vi "Perform_Math_Main.vi"(0 "Input_1":dbl caption="Input1", 5 "Input_2":dbl caption="Input2", 11 "Error_In":errorcluster) -> (4 "Output":dbl, 15 "Error_Out":errorcluster)   [LabVIEW 2023]
doc: "This is the main vi which Performs Math calculations using CDLL and .Net DLL."
uses:
  Controls/Operation.ctl
  Controls/DLL_Type.ctl
  D:/Project Git file/Assignments/Assignment-11/Assignment-11_LV23V/Build_.Net_Dll/Perform_Math_Assembly.dll
  Build_.Net_Dll/Perform_Math_Assembly.dll
  Build_Dll/Perform_Math.dll
panel:
  in  "DLL_Type":T1
  in  "Operation":T2
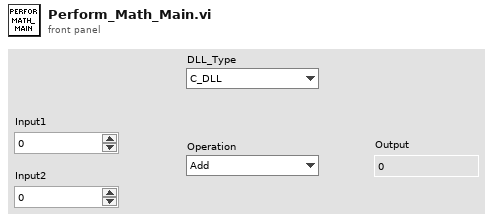
[diagram p1: front panel]
types:
  T1 = typedef "DLL_Type.ctl" = enum16{"C_DLL", ".NET_DLL"}
  T2 = typedef "Operation.ctl" = enum16{"Add", "Sub", "Mul", "Div"}
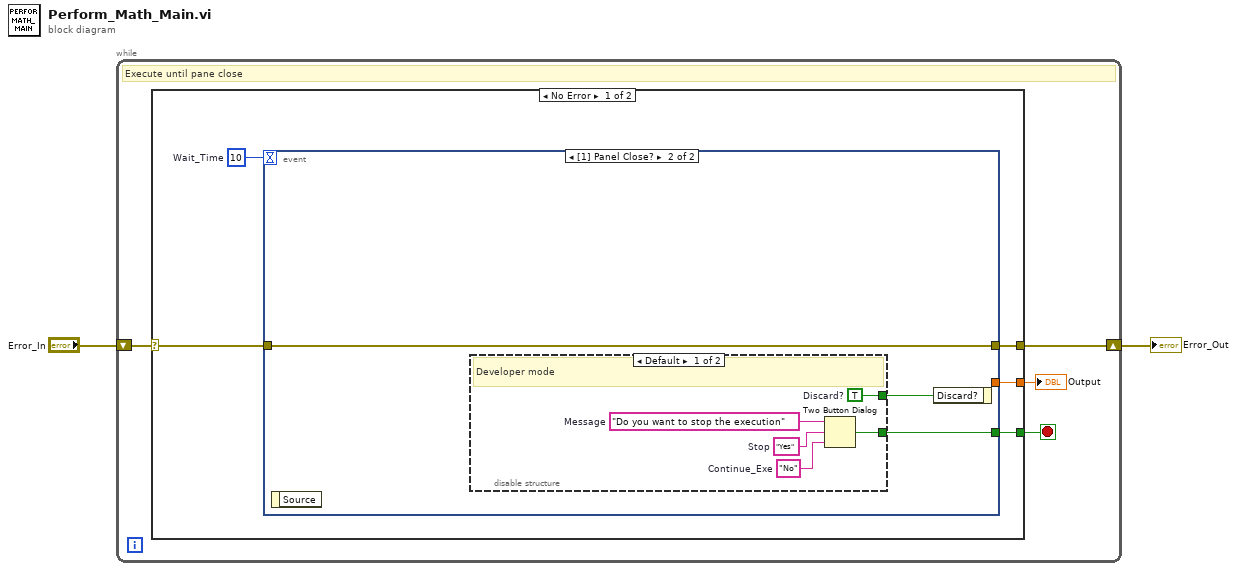
[diagram p0: block diagram]
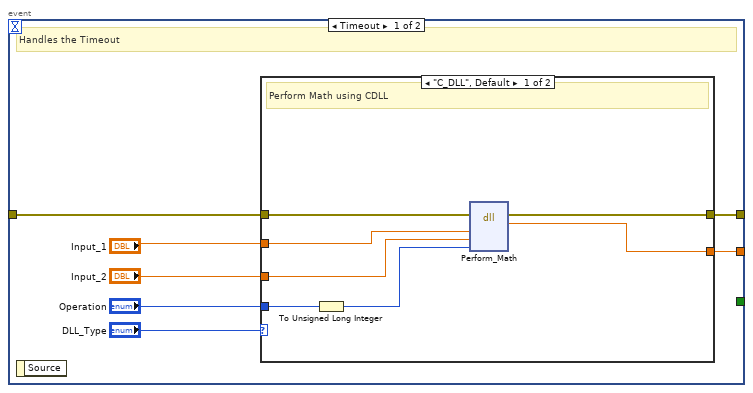
[diagram p2: hidden frame]
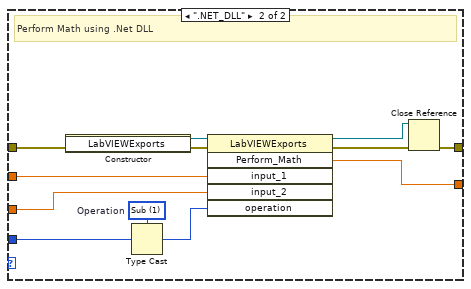
[diagram p3: hidden frame]
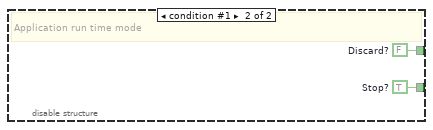
[diagram p4: hidden frame]
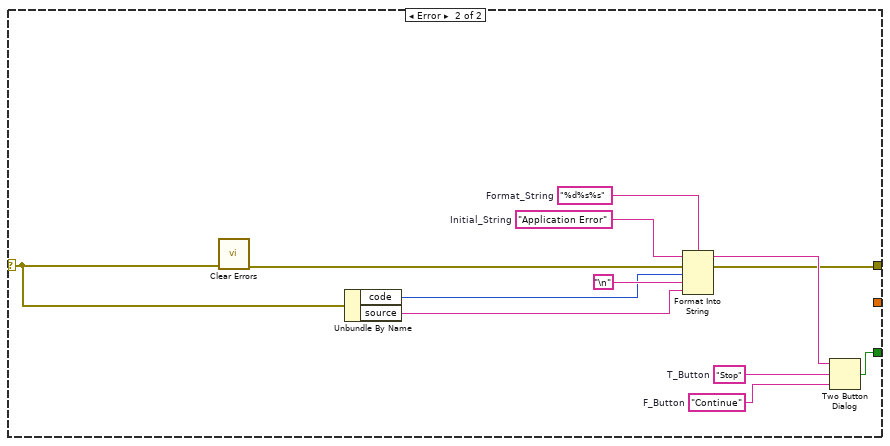
[diagram p5: hidden frame]
diagram:
  n1 = while {
    shift-right: [w5] -> w1
    shift-left: "Error_In" -> [w6]
    stop <- w3 stop-if-true
    # "Execute until pane close"
    n2 = case shown="No Error" w6 {
      selector: w6 -> [w11 w50]
      tunnel: [w10 w49] -> w5
      tunnel: [w9 _] -> w4
      tunnel: [w7 w48] -> w3
      frame No Error {
        w8 = 10  # Wait_Time
        n3 = event shown="[1] Panel Close?" {
          selector: _ -> [_ _]
          dyn-events: _ -> [_ _]
          timeout: w8 -> [_ _]
          tunnel: w11 -> [w18 w40]
          tunnel: [w17 w40] -> w10
          tunnel: [w14 _] -> w9
          tunnel: [_ w38] -> w7
          event Timeout {
            # "Handles the Timeout"
            n4 = event-data() -> ()  [unwired: 1 in, 1 out]
            n5 = case shown="\"C_DLL\", Default" "DLL_Type" {
              tunnel: w18 -> [w25 w37]
              tunnel: [w24 w27] -> w17
              tunnel: "Input_1" -> [w23 w33]
              tunnel: "Input_2" -> [w22 w32]
              tunnel: [w21 w34] -> w14
              tunnel: "Operation" -> [w20 w30]
              frame "C_DLL", Default {
                # "Perform Math using CDLL"
                n6 = To Unsigned Long Integer(number=w20) -> (unsigned 32bit integer=w19:u32)
                n7 = dll-call lib="D:/Project Git file/Assignments/Assignment-11/Assignment-11_LV23V/Build_Dll/Perform_Math.dll" fn="Perform_Math"(error in=w25, "Input_1"=w23, "Input_2"=w22, "Operation"=w19) -> (error out=w24:errorcluster, "return type"=w21:dbl)  [unwired: 5 in, 1 out]
              }
              frame ".NET_DLL" {
                w31 = u16 1 items=["Add", "Sub", "Mul", "Div"]  # Operation
                # "Perform Math using .Net DLL"
                n8 = constructor class="LabVIEWExports" ("Constructor Node")(error in=w37) -> (reference out=w35:refnum<k24>, error out=w36:errorcluster)  [unwired: 2 in, 1 out]
                n9 = Type Cast(type=w31, x=w30) -> (*(type *) &x=w29:u16)
                n10 = invoke on="Invoke Node" class="LabVIEWExports" method="Perform_Math"(reference=w35, error in=w36, "input_1"=w33, "input_2"=w32, "operation"=w29) -> (reference out=w26:refnum<k24>, error out=w28:errorcluster, "Perform_Math"=w34:dbl)  [unwired: 1 in, 3 out]
                n11 = Close Reference(reference=w26, error in (no error)=w28) -> (error out=w27:errorcluster)
              }
            }
          }
          event Panel Close? {
            n12 = event-data() -> ()  [unwired: 1 in, 1 out]
            n13 = disable-structure shown="Default" {
              disable-tunnel: [w42 w46] -> w38
              disable-tunnel: [w41 w47] -> w39
              frame condition #0 (active) {
                w41 = TRUE  # Discard?
                w43 = "No"  # Continue_Exe
                w44 = "Yes"  # Stop
                w45 = "Do you want to stop the execution"  # Message
                # "Developer mode"
                n14 = Two Button Dialog(message=w45, 1:w43, 2:w44) -> (T button?=w42:bool)
              }
              frame condition #1 {
                w46 = TRUE  # Stop?
                w47 = FALSE  # Discard?
                # "Application run time mode"
              }
            }
            n15 = event-data ("Event Filter Node")("Discard?"=w39) -> ()  [unwired: 1 in, 1 out]
          }
        }
      }
      frame Error {
        w55 = "%d%s%s"  # Format_String
        w56 = "Application Error"  # Initial_String
        w57 = "Stop"  # T_Button
        w58 = "Continue"  # F_Button
        n16 = call <vilib>:"Clear Errors.vi"("error in (no error)"=w50) -> ("error out"=w53:errorcluster)  [unwired: 5 in, 1 out]
        n17 = Unbundle By Name(w50) -> ("code"=w52:i32, "source"=w51:string)
        n18 = Format Into String(format string=w55, initial string=w56, error in=w53, w52, "\n" ("Line Feed Constant"), w51) -> (resulting string=w59:string, error out=w49:errorcluster)
        n19 = Two Button Dialog(message=w59, 1:w58, 2:w57) -> (T button?=w48:bool)
      }
    }
    "Output" <- w4
  }
  "Error_Out" <- w1
